vi "Load CSV.vi"(0 "CSV Path":path) -> (10 "Header":string[](array[string]), 11 "error out":errorcluster, 12 "CSV Array":string[][](array[string]), 13 "indices":T1, 14 "Fuel":string[](array[string]), 15 "Oxidizer":string[](array[string]), 16 "Initial Pressure":string[](array[string]), 17 "Equivalence Ratio":string[](array[string]), 18 "Diluent":string[](array[string]), 19 "Diluent Mole Fraction":string[](array[string]))   [LabVIEW 2018]
uses:
  <vilib>/Utility/file.llb/Read Delimited Spreadsheet (string).vi
  Sort 1D Array sub vis/Sort 1D String.vi
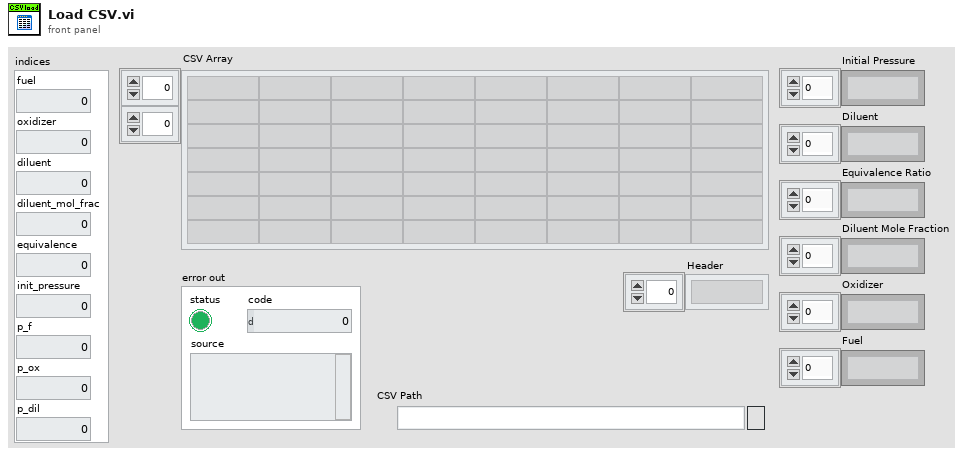
[diagram p1: front panel]
types:
  T1 = cluster{"fuel":i32, "oxidizer":i32, "diluent":i32, "diluent_mol_frac":i32, "equivalence":i32, "init_pressure":i32, "p_f":i32, "p_ox":i32, "p_dil":i32}
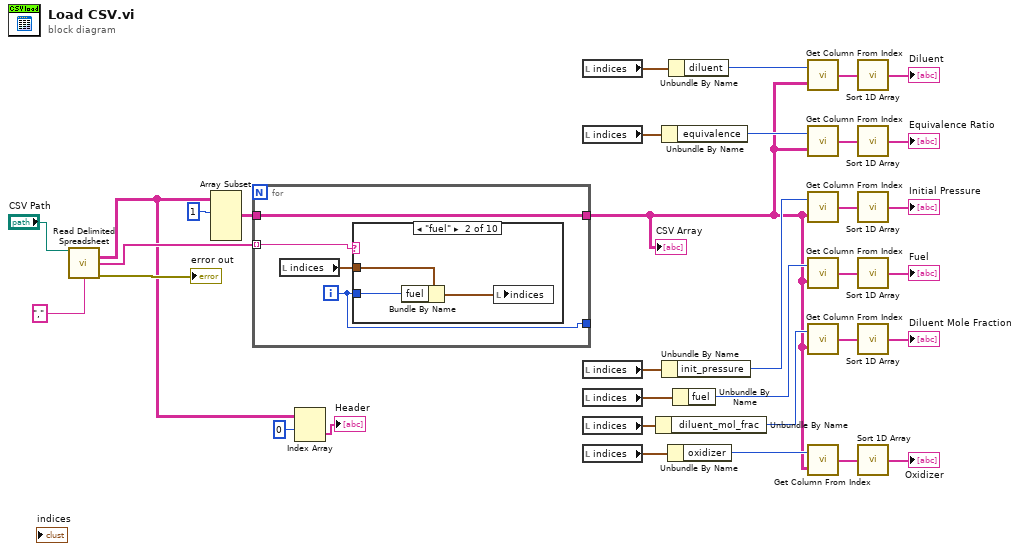
[diagram p0: block diagram]
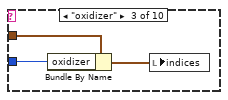
[diagram p3: hidden frame]
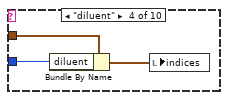
[diagram p4: hidden frame]
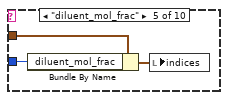
[diagram p5: hidden frame]
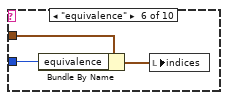
[diagram p6: hidden frame]
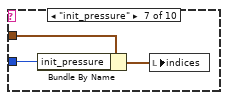
[diagram p7: hidden frame]
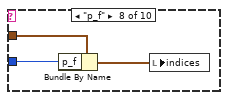
[diagram p8: hidden frame]
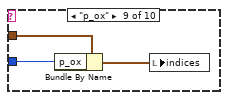
[diagram p9: hidden frame]
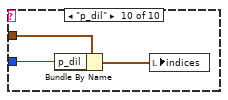
[diagram p10: hidden frame]
diagram:
  n1 = call-poly <vilib>:"Read Delimited Spreadsheet.vi"("file path (dialog if empty)"="CSV Path", "delimiter (\\t)"="," ("delimiter (\\t)")) -> ("all rows"=w4:string[][], "first row"=w32:string[], "error out"=→"error out":errorcluster)  [unwired: 8 in, 3 out]
  n2 = Array Subset(array=w4, index (row)=1 ("index")) -> (w28:string[][])  [unwired: 3 in]
  n3 = for {
    tunnel: w32 -> [w38] mode=indexing
    tunnel: [w37] -> _
    tunnel: w28 -> [w35]
    tunnel: [w35] -> w12
    i -> [w37]
    n4 = local read "indices"() -> (w36:T1)
    n5 = case shown="\"fuel\"" w38 {
      tunnel: w36 -> [_ w41 w42 w45 w49 w52 w54 w58 w60 w63]
      tunnel: w37 -> [_ w40 w44 w46 w48 w51 w55 w57 w61 w64]
      frame Default {
      }
      frame "fuel" {
        n6 = Bundle By Name(cluster=w41, "fuel"=w40) -> (w39:T1)
        n7 = local write "indices"(w39) -> ()
      }
      frame "oxidizer" {
        n8 = Bundle By Name(cluster=w42, "oxidizer"=w44) -> (w43:T1)
        n9 = local write "indices"(w43) -> ()
      }
      frame "diluent" {
        n10 = Bundle By Name(cluster=w45, "diluent"=w46) -> (w47:T1)
        n11 = local write "indices"(w47) -> ()
      }
      frame "diluent_mol_frac" {
        n12 = Bundle By Name(cluster=w49, "diluent_mol_frac"=w48) -> (w50:T1)
        n13 = local write "indices"(w50) -> ()
      }
      frame "equivalence" {
        n14 = Bundle By Name(cluster=w52, "equivalence"=w51) -> (w53:T1)
        n15 = local write "indices"(w53) -> ()
      }
      frame "init_pressure" {
        n16 = Bundle By Name(cluster=w54, "init_pressure"=w55) -> (w56:T1)
        n17 = local write "indices"(w56) -> ()
      }
      frame "p_f" {
        n18 = Bundle By Name(cluster=w58, "p_f"=w57) -> (w59:T1)
        n19 = local write "indices"(w59) -> ()
      }
      frame "p_ox" {
        n20 = Bundle By Name(cluster=w60, "p_ox"=w61) -> (w62:T1)
        n21 = local write "indices"(w62) -> ()
      }
      frame "p_dil" {
        n22 = Bundle By Name(cluster=w63, "p_dil"=w64) -> (w65:T1)
        n23 = local write "indices"(w65) -> ()
      }
    }
  }
  "CSV Array" <- w12
  n24 = Index Array(array=w4, index (row)=0) -> (element=→"Header":string[])  [unwired: 1 in]
  n25 = local read "indices"() -> (w23:T1)
  n26 = local read "indices"() -> (w20:T1)
  n27 = local read "indices"() -> (w26:T1)
  n28 = local read "indices"() -> (w30:T1)
  n29 = local read "indices"() -> (w17:T1)
  n30 = local read "indices"() -> (w14:T1)
  n31 = Unbundle By Name(w17) -> ("diluent_mol_frac"=w16:i32)
  n32 = Unbundle By Name(w20) -> ("equivalence"=w21:i32)
  n33 = Unbundle By Name(w26) -> ("init_pressure"=w27:i32)
  n34 = Unbundle By Name(w14) -> ("oxidizer"=w15:i32)
  n35 = Unbundle By Name(w23) -> ("diluent"=w22:i32)
  n36 = Unbundle By Name(w30) -> ("fuel"=w29:i32)
  n37 = call "Get Column From Index.vi"("array"=w12, "index"=w22) -> ("subarray"=w24:string[])
  n38 = call "Get Column From Index.vi"("array"=w12, "index"=w21) -> ("subarray"=w19:string[])
  n39 = call "Get Column From Index.vi"("array"=w12, "index"=w27) -> ("subarray"=w25:string[])
  n40 = call "Get Column From Index.vi"("array"=w12, "index"=w29) -> ("subarray"=w31:string[])
  n41 = call "Get Column From Index.vi"("array"=w12, "index"=w16) -> ("subarray"=w18:string[])
  n42 = call "Get Column From Index.vi"("array"=w12, "index"=w15) -> ("subarray"=w13:string[])
  n43 = call-poly "Sort 1D Array.vi"("1D input array"=w24) -> ("output array"=→"Diluent":string[])
  n44 = call-poly "Sort 1D Array.vi"("1D input array"=w19) -> ("output array"=→"Equivalence Ratio":string[])
  n45 = call-poly "Sort 1D Array.vi"("1D input array"=w25) -> ("output array"=→"Initial Pressure":string[])
  n46 = call-poly "Sort 1D Array.vi"("1D input array"=w31) -> ("output array"=→"Fuel":string[])
  n47 = call-poly "Sort 1D Array.vi"("1D input array"=w18) -> ("output array"=→"Diluent Mole Fraction":string[])
  n48 = call-poly "Sort 1D Array.vi"("1D input array"=w13) -> ("output array"=→"Oxidizer":string[])
